vi "Slope Calibration Sampling Frequency.vi"() -> (0 "Sampling Frequency":dbl)   [LabVIEW 2013]
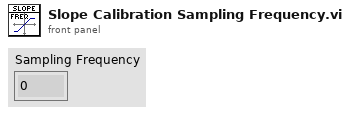
[diagram p1: front panel]
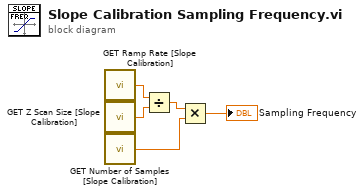
[diagram p0: block diagram]
diagram:
  n1 = call "GET Ramp Rate [Slope Calibration].vi"() -> ("Ramp Rate"=w2:dbl)
  n2 = call "GET Z Scan Size [Slope Calibration].vi"() -> ("Z Scan Size"=w1:dbl)
  n3 = call "GET Number of Samples [Slope Calibration].vi"() -> ("Number of Samples"=w4:dbl)
  n4 = Divide(x=w2, y=w1) -> (x/y=w3:dbl)
  n5 = Multiply(x=w3, y=w4) -> (x*y=→"Sampling Frequency":dbl)
